vi "pp2_DAQwriteDO.vi"(8 "error in (no error)":errorcluster, 10 "Daq config":T1={"Sound AO"="Dev2/ao0", "Shock intesity AO"="Dev1/ao1", "Code/LED DO"="Dev1/port1:2", "Switches DI"="Dev1/port0/line0:1", "Webcam"="cam0", "Sound AO task"="", "Sound card task"=0, "Shock intensity AO task"="", "Code/LED DO task"="", "Switch DI task"="", "AO <=> Sound card"=FALSE, "Sound card"=0, "sample rate"=8000.0, "Variable shock"=FALSE, "Webcam on"=FALSE, "Tone gate PFI"="/Dev1/PFI1"} {"sample rate" min=8000.0; "Sound card task" format="%.0x"}, 11 "DAQ Digital In":u16 format="%b") -> (0 "error out":errorcluster, 2 "Daq config 2":T1={"Sound AO"="Dev2/ao0", "Shock intesity AO"="Dev1/ao1", "Code/LED DO"="Dev1/port1:2", "Switches DI"="Dev1/port0/line0:1", "Webcam"="cam0", "Sound AO task"="", "Sound card task"=0, "Shock intensity AO task"="", "Code/LED DO task"="", "Switch DI task"="", "AO <=> Sound card"=FALSE, "Sound card"=0, "sample rate"=8000.0, "Variable shock"=FALSE, "Webcam on"=FALSE, "Tone gate PFI"="/Dev1/PFI1"} {"sample rate" min=8000.0; "Sound card task" format="%.0x"})   [LabVIEW 2013]
uses:
  pp2_CTL_DaqConfig.ctl
  <vilib>/userdefined/High Color/IMAQdx.ctl
  <vilib>/sound2/lvsound2.llb/Sound Output Task ID.ctl
  <vilib>/DAQmx/write.llb/DAQmx Write (Digital 1D U16 1Chan NSamp).vi
  <vilib>/DAQmx/miscellaneous.llb/DAQmx Fill In Error Info.vi
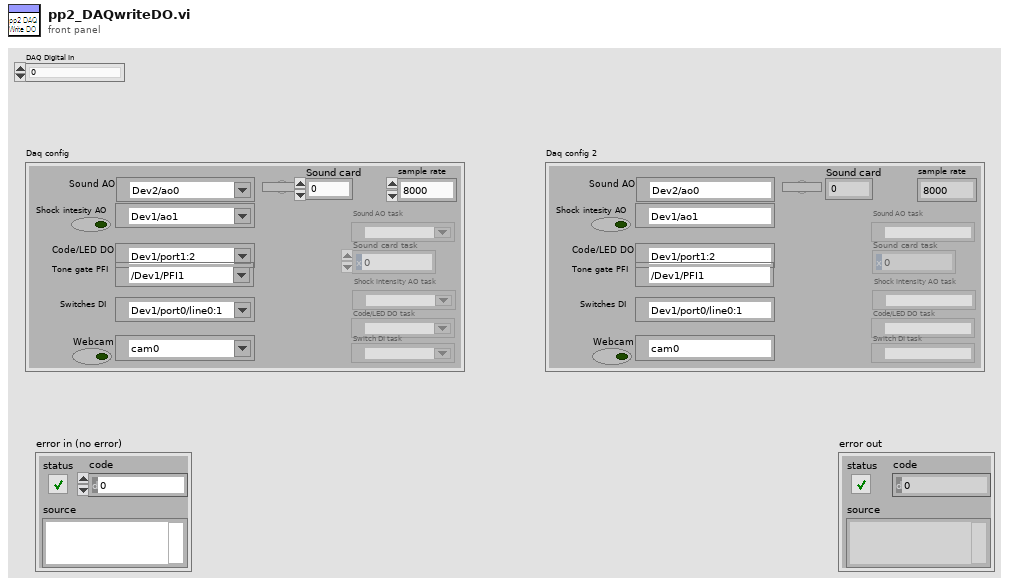
[diagram p1: front panel]
types:
  T1 = typedef "pp2_CTL_DaqConfig.ctl" = cluster{"Sound AO":tag, "Shock intesity AO":tag, "Code/LED DO":tag, "Switches DI":tag, "Webcam":T2, "Sound AO task":refnum<k21>, "Sound card task":T3, "Shock intensity AO task":refnum<k21>, "Code/LED DO task":refnum<k21>, "Switch DI task":refnum<k21>, "AO <=> Sound card":bool, "Sound card":u32, "sample rate":dbl, "Variable shock":bool, "Webcam on":bool, "Tone gate PFI":tag}
  T2 = typedef "IMAQdx.ctl" = refnum<k21>
  T3 = typedef "Sound Output Task ID.ctl" = u32
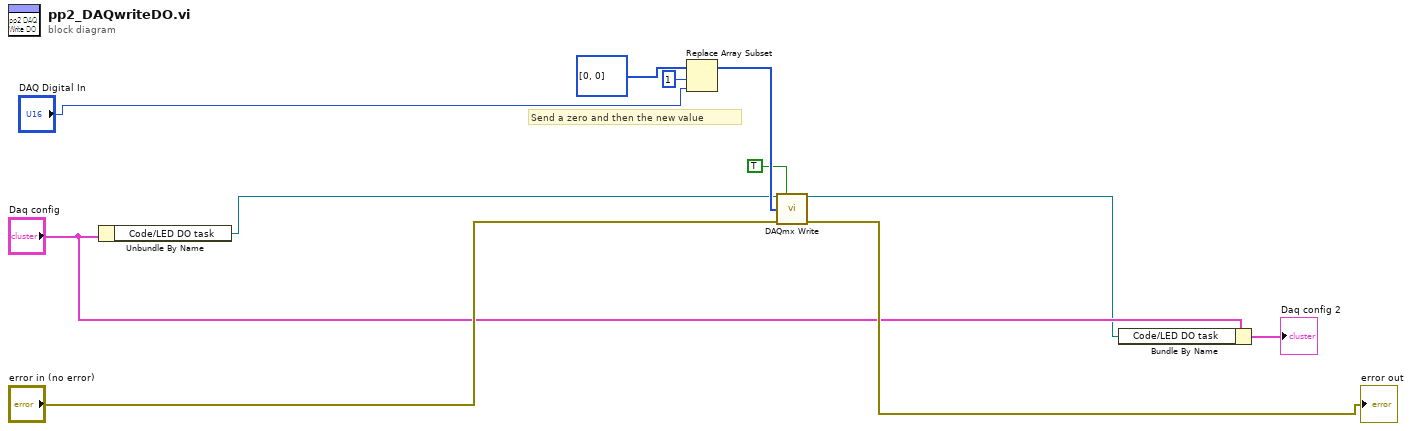
[diagram p0: block diagram]
diagram:
  # "Send a zero and then the new value"
  n1 = Unbundle By Name("Daq config") -> ("Code/LED DO task"=w5:refnum<k21>)
  n2 = Replace Array Subset(array=u16[] [0, 0] ("data"), new element="DAQ Digital In", index=1) -> (w7:u16[])
  n3 = call-poly <vilib>:"DAQmx Write.vi"("task/channels in"=w5, "auto start"=TRUE, "data"=w7, "error in"="error in (no error)") -> ("task out"=w1:refnum<k21>, "error out"=→"error out":errorcluster)  [unwired: 9 in, 1 out]
  n4 = Bundle By Name(cluster="Daq config", "Code/LED DO task"=w1) -> (→"Daq config 2":T1)
